vi "CRYO_LeakTest_tmp.vi"() -> ()   [LabVIEW 2017]
uses:
  USBData.lvclass
panel:
  in  "Stop Button":bool
  out "Cycle #":u32=37
  out "Time of Last Measurement":timestamp=timestamp(3679441672.677524 s since 1904-01-01)
  in  "wait (ms)":u32=1000
  in  "?":enum32{"CONFIG", "MEASUREMENT"}(tab)=enum."MEASUREMENT"
  in  "USBSettings":T1(array[cluster])=[{"Label"="0", "FileFormat"="%2.2f", "Physical CH"="Dev2/ai0", "ConversionType"={"Type"=enum."CC-10_LOG", "ConversionParameters"=[0.5, 9.0]}, "VoltageLimits"=[0.0, 10.0]}, {"Label"="1", "FileFormat"="%2.2f", "Physical CH"="Dev2/ai1", "ConversionType"={"Type"=enum."LeakDet_EXP", "ConversionParameters"=[0.0, 1.0]}, "VoltageLimits"=[0.0, 10.0]}, {"Label"="2", "FileFormat"="%2.2f", "Physical CH"="Dev2/ai2", "ConversionType"={"Type"=enum."LeakDet_Mantissa", "ConversionParameters"=[0.0, 1.0]}, "VoltageLimits"=[0.0, 10.0]}, {"Label"="3", "FileFormat"="%2.2f", "Physical CH"="Dev2/ai3", "ConversionType"={"Type"=enum."SimpleProp", "ConversionParameters"=[0.0, 1.0]}, "VoltageLimits"=[0.0, 10.0]}]
  in  "RUN identifier":string="TEST"
  in  "Base Path":path=path "C:/LabVIEW/DATA/TestData/TestSeries"
  in  "Activate":bool=TRUE
  out "error out":errorcluster
  in  "InstName":string="USB6210"
  out "Status":T2(ring)=enum."Waiting"
  out "Waveform Chart 2":dbl(graph)
  out "Waveform Chart":dbl(graph)
  out "LeakRate":dbl=7.334292864367354e-09 format="%_3e"
  in  "Take Screenshot! 1":bool
  in  "Screenshot suffix 1":string="Graph1"
  in  "log/linear 2":bool=TRUE
  in  "Plot in \nGraph2?":bool[](array[boolean])=[TRUE, TRUE, FALSE, FALSE, FALSE, FALSE]
  out "Graph 2":T3(graph)=[{"TimeArray"=[timestamp(3679441636.668932 s since 1904-01-01), timestamp(3679441637.669246 s since 1904-01-01), timestamp(3679441638.668856 s since 1904-01-01), timestamp(3679441639.6687136 s since 1904-01-01), timestamp(3679441640.6689286 s since 1904-01-01), timestamp(3679441641.669116 s since 1904-01-01), timestamp(3679441642.6704025 s since 1904-01-01), timestamp(3679441643.6717186 s since 1904-01-01), timestamp(3679441644.671928 s since 1904-01-01), timestamp(3679441645.6718183 s since 1904-01-01), timestamp(3679441646.6721153 s since 1904-01-01), timestamp(3679441647.672172 s since 1904-01-01), timestamp(3679441648.672178 s since 1904-01-01), timestamp(3679441649.672041 s since 1904-01-01), timestamp(3679441650.6726017 s since 1904-01-01), timestamp(3679441651.6730194 s since 1904-01-01), timestamp(3679441652.673001 s since 1904-01-01), timestamp(3679441653.6726832 s since 1904-01-01), timestamp(3679441654.673409 s since 1904-01-01), timestamp(3679441655.6734624 s since 1904-01-01), timestamp(3679441656.674424 s since 1904-01-01), timestamp(3679441657.675055 s since 1904-01-01), timestamp(3679441658.674728 s since 1904-01-01), timestamp(3679441659.6749954 s since 1904-01-01), timestamp(3679441660.6749263 s since 1904-01-01), timestamp(3679441661.6754694 s since 1904-01-01), timestamp(3679441662.6761866 s since 1904-01-01), timestamp(3679441663.675552 s since 1904-01-01), timestamp(3679441664.675677 s since 1904-01-01), timestamp(3679441665.6756015 s since 1904-01-01), timestamp(3679441666.675688 s since 1904-01-01), timestamp(3679441667.6754055 s since 1904-01-01), timestamp(3679441668.6766486 s since 1904-01-01), timestamp(3679441669.677348 s since 1904-01-01), timestamp(3679441670.6767225 s since 1904-01-01), timestamp(3679441671.6770015 s since 1904-01-01), timestamp(3679441672.677524 s since 1904-01-01)], "DataArray"=[70.50247496839857, -9.0, 4.487131051293313, 0.0]}, {"TimeArray"=[timestamp(3679441636.668932 s since 1904-01-01), timestamp(3679441637.669246 s since 1904-01-01), timestamp(3679441638.668856 s since 1904-01-01), timestamp(3679441639.6687136 s since 1904-01-01), timestamp(3679441640.6689286 s since 1904-01-01), timestamp(3679441641.669116 s since 1904-01-01), timestamp(3679441642.6704025 s since 1904-01-01), timestamp(3679441643.6717186 s since 1904-01-01), timestamp(3679441644.671928 s since 1904-01-01), timestamp(3679441645.6718183 s since 1904-01-01), timestamp(3679441646.6721153 s since 1904-01-01), timestamp(3679441647.672172 s since 1904-01-01), timestamp(3679441648.672178 s since 1904-01-01), timestamp(3679441649.672041 s since 1904-01-01), timestamp(3679441650.6726017 s since 1904-01-01), timestamp(3679441651.6730194 s since 1904-01-01), timestamp(3679441652.673001 s since 1904-01-01), timestamp(3679441653.6726832 s since 1904-01-01), timestamp(3679441654.673409 s since 1904-01-01), timestamp(3679441655.6734624 s since 1904-01-01), timestamp(3679441656.674424 s since 1904-01-01), timestamp(3679441657.675055 s since 1904-01-01), timestamp(3679441658.674728 s since 1904-01-01), timestamp(3679441659.6749954 s since 1904-01-01), timestamp(3679441660.6749263 s since 1904-01-01), timestamp(3679441661.6754694 s since 1904-01-01), timestamp(3679441662.6761866 s since 1904-01-01), timestamp(3679441663.675552 s since 1904-01-01), timestamp(3679441664.675677 s since 1904-01-01), timestamp(3679441665.6756015 s since 1904-01-01), timestamp(3679441666.675688 s since 1904-01-01), timestamp(3679441667.6754055 s since 1904-01-01), timestamp(3679441668.6766486 s since 1904-01-01), timestamp(3679441669.677348 s since 1904-01-01), timestamp(3679441670.6767225 s since 1904-01-01), timestamp(3679441671.6770015 s since 1904-01-01), timestamp(3679441672.677524 s since 1904-01-01)], "DataArray"=[70.45978396050337, -9.0, 5.396766437487628, 0.0]}, {"TimeArray"=[timestamp(3679441636.668932 s since 1904-01-01), timestamp(3679441637.669246 s since 1904-01-01), timestamp(3679441638.668856 s since 1904-01-01), timestamp(3679441639.6687136 s since 1904-01-01), timestamp(3679441640.6689286 s since 1904-01-01), timestamp(3679441641.669116 s since 1904-01-01), timestamp(3679441642.6704025 s since 1904-01-01), timestamp(3679441643.6717186 s since 1904-01-01), timestamp(3679441644.671928 s since 1904-01-01), timestamp(3679441645.6718183 s since 1904-01-01), timestamp(3679441646.6721153 s since 1904-01-01), timestamp(3679441647.672172 s since 1904-01-01), timestamp(3679441648.672178 s since 1904-01-01), timestamp(3679441649.672041 s since 1904-01-01), timestamp(3679441650.6726017 s since 1904-01-01), timestamp(3679441651.6730194 s since 1904-01-01), timestamp(3679441652.673001 s since 1904-01-01), timestamp(3679441653.6726832 s since 1904-01-01), timestamp(3679441654.673409 s since 1904-01-01), timestamp(3679441655.6734624 s since 1904-01-01), timestamp(3679441656.674424 s since 1904-01-01), timestamp(3679441657.675055 s since 1904-01-01), timestamp(3679441658.674728 s since 1904-01-01), timestamp(3679441659.6749954 s since 1904-01-01), timestamp(3679441660.6749263 s since 1904-01-01), timestamp(3679441661.6754694 s since 1904-01-01), timestamp(3679441662.6761866 s since 1904-01-01), timestamp(3679441663.675552 s since 1904-01-01), timestamp(3679441664.675677 s since 1904-01-01), timestamp(3679441665.6756015 s since 1904-01-01), timestamp(3679441666.675688 s since 1904-01-01), timestamp(3679441667.6754055 s since 1904-01-01), timestamp(3679441668.6766486 s since 1904-01-01), timestamp(3679441669.677348 s since 1904-01-01), timestamp(3679441670.6767225 s since 1904-01-01), timestamp(3679441671.6770015 s since 1904-01-01), timestamp(3679441672.677524 s since 1904-01-01)], "DataArray"=[70.11918514591878, -9.0, 6.016059802087263, 0.0]}, {"TimeArray"=[timestamp(3679441636.668932 s since 1904-01-01), timestamp(3679441637.669246 s since 1904-01-01), timestamp(3679441638.668856 s since 1904-01-01), timestamp(3679441639.6687136 s since 1904-01-01), timestamp(3679441640.6689286 s since 1904-01-01), timestamp(3679441641.669116 s since 1904-01-01), timestamp(3679441642.6704025 s since 1904-01-01), timestamp(3679441643.6717186 s since 1904-01-01), timestamp(3679441644.671928 s since 1904-01-01), timestamp(3679441645.6718183 s since 1904-01-01), timestamp(3679441646.6721153 s since 1904-01-01), timestamp(3679441647.672172 s since 1904-01-01), timestamp(3679441648.672178 s since 1904-01-01), timestamp(3679441649.672041 s since 1904-01-01), timestamp(3679441650.6726017 s since 1904-01-01), timestamp(3679441651.6730194 s since 1904-01-01), timestamp(3679441652.673001 s since 1904-01-01), timestamp(3679441653.6726832 s since 1904-01-01), timestamp(3679441654.673409 s since 1904-01-01), timestamp(3679441655.6734624 s since 1904-01-01), timestamp(3679441656.674424 s since 1904-01-01), timestamp(3679441657.675055 s since 1904-01-01), timestamp(3679441658.674728 s since 1904-01-01), timestamp(3679441659.6749954 s since 1904-01-01), timestamp(3679441660.6749263 s since 1904-01-01), timestamp(3679441661.6754694 s since 1904-01-01), timestamp(3679441662.6761866 s since 1904-01-01), timestamp(3679441663.675552 s since 1904-01-01), timestamp(3679441664.675677 s since 1904-01-01), timestamp(3679441665.6756015 s since 1904-01-01), timestamp(3679441666.675688 s since 1904-01-01), timestamp(3679441667.6754055 s since 1904-01-01), timestamp(3679441668.6766486 s since 1904-01-01), timestamp(3679441669.677348 s since 1904-01-01), timestamp(3679441670.6767225 s since 1904-01-01), timestamp(3679441671.6770015 s since 1904-01-01), timestamp(3679441672.677524 s since 1904-01-01)], "DataArray"=[75.51986553242087, -9.0, 6.43017264767335, 0.0]}, {"TimeArray"=[timestamp(3679441636.668932 s since 1904-01-01), timestamp(3679441637.669246 s since 1904-01-01), timestamp(3679441638.668856 s since 1904-01-01), timestamp(3679441639.6687136 s since 1904-01-01), timestamp(3679441640.6689286 s since 1904-01-01), timestamp(3679441641.669116 s since 1904-01-01), timestamp(3679441642.6704025 s since 1904-01-01), timestamp(3679441643.6717186 s since 1904-01-01), timestamp(3679441644.671928 s since 1904-01-01), timestamp(3679441645.6718183 s since 1904-01-01), timestamp(3679441646.6721153 s since 1904-01-01), timestamp(3679441647.672172 s since 1904-01-01), timestamp(3679441648.672178 s since 1904-01-01), timestamp(3679441649.672041 s since 1904-01-01), timestamp(3679441650.6726017 s since 1904-01-01), timestamp(3679441651.6730194 s since 1904-01-01), timestamp(3679441652.673001 s since 1904-01-01), timestamp(3679441653.6726832 s since 1904-01-01), timestamp(3679441654.673409 s since 1904-01-01), timestamp(3679441655.6734624 s since 1904-01-01), timestamp(3679441656.674424 s since 1904-01-01), timestamp(3679441657.675055 s since 1904-01-01), timestamp(3679441658.674728 s since 1904-01-01), timestamp(3679441659.6749954 s since 1904-01-01), timestamp(3679441660.6749263 s since 1904-01-01), timestamp(3679441661.6754694 s since 1904-01-01), timestamp(3679441662.6761866 s since 1904-01-01), timestamp(3679441663.675552 s since 1904-01-01), timestamp(3679441664.675677 s since 1904-01-01), timestamp(3679441665.6756015 s since 1904-01-01), timestamp(3679441666.675688 s since 1904-01-01), timestamp(3679441667.6754055 s since 1904-01-01), timestamp(3679441668.6766486 s since 1904-01-01), timestamp(3679441669.677348 s since 1904-01-01), timestamp(3679441670.6767225 s since 1904-01-01), timestamp(3679441671.6770015 s since 1904-01-01), timestamp(3679441672.677524 s since 1904-01-01)], "DataArray"=[72.7584215196649, -9.0, 6.711377973370896, 0.0]}, {"TimeArray"=[timestamp(3679441636.668932 s since 1904-01-01), timestamp(3679441637.669246 s since 1904-01-01), timestamp(3679441638.668856 s since 1904-01-01), timestamp(3679441639.6687136 s since 1904-01-01), timestamp(3679441640.6689286 s since 1904-01-01), timestamp(3679441641.669116 s since 1904-01-01), timestamp(3679441642.6704025 s since 1904-01-01), timestamp(3679441643.6717186 s since 1904-01-01), timestamp(3679441644.671928 s since 1904-01-01), timestamp(3679441645.6718183 s since 1904-01-01), timestamp(3679441646.6721153 s since 1904-01-01), timestamp(3679441647.672172 s since 1904-01-01), timestamp(3679441648.672178 s since 1904-01-01), timestamp(3679441649.672041 s since 1904-01-01), timestamp(3679441650.6726017 s since 1904-01-01), timestamp(3679441651.6730194 s since 1904-01-01), timestamp(3679441652.673001 s since 1904-01-01), timestamp(3679441653.6726832 s since 1904-01-01), timestamp(3679441654.673409 s since 1904-01-01), timestamp(3679441655.6734624 s since 1904-01-01), timestamp(3679441656.674424 s since 1904-01-01), timestamp(3679441657.675055 s since 1904-01-01), timestamp(3679441658.674728 s since 1904-01-01), timestamp(3679441659.6749954 s since 1904-01-01), timestamp(3679441660.6749263 s since 1904-01-01), timestamp(3679441661.6754694 s since 1904-01-01), timestamp(3679441662.6761866 s since 1904-01-01), timestamp(3679441663.675552 s since 1904-01-01), timestamp(3679441664.675677 s since 1904-01-01), timestamp(3679441665.6756015 s since 1904-01-01), timestamp(3679441666.675688 s since 1904-01-01), timestamp(3679441667.6754055 s since 1904-01-01), timestamp(3679441668.6766486 s since 1904-01-01), timestamp(3679441669.677348 s since 1904-01-01), timestamp(3679441670.6767225 s since 1904-01-01), timestamp(3679441671.6770015 s since 1904-01-01), timestamp(3679441672.677524 s since 1904-01-01)], "DataArray"=[4.487131051293314e-09, 5.396766437487628e-09, 6.016059802087263e-09, 6.430172647673351e-09, 6.711377973370896e-09, 6.899791063470254e-09, 7.023690049144573e-09, 7.123059208849688e-09, 7.183956553663248e-09, 7.2279525979897775e-09, 7.25754635696336e-09, 7.2743819199666565e-09, 7.285430259185793e-09, 7.2907571374582694e-09, 7.29884610085954e-09, 7.306737772921106e-09, 7.30930256649171e-09, 7.3202851443231995e-09, 7.326138135237289e-09, 7.323441813920113e-09, 7.328834456885956e-09, 7.325283203914373e-09, 7.331201958895281e-09, 7.326861538535115e-09, 7.330807375263062e-09, 7.33231994614466e-09, 7.3306758473074275e-09, 7.326664246703097e-09, 7.3291632766052906e-09, 7.335082031766526e-09, 7.332911821527113e-09, 7.3328460575291335e-09, 7.333174877285675e-09, 7.337844117606753e-09, 7.332451473872307e-09, 7.335279323589255e-09, 7.334292864367354e-09]}] caption="XY Graph"
  out "Graph 1":T4(graph)=[{"TimeArray"=[timestamp(3679441636.668932 s since 1904-01-01), timestamp(3679441637.669246 s since 1904-01-01), timestamp(3679441638.668856 s since 1904-01-01), timestamp(3679441639.6687136 s since 1904-01-01), timestamp(3679441640.6689286 s since 1904-01-01), timestamp(3679441641.669116 s since 1904-01-01), timestamp(3679441642.6704025 s since 1904-01-01), timestamp(3679441643.6717186 s since 1904-01-01), timestamp(3679441644.671928 s since 1904-01-01), timestamp(3679441645.6718183 s since 1904-01-01), timestamp(3679441646.6721153 s since 1904-01-01), timestamp(3679441647.672172 s since 1904-01-01), timestamp(3679441648.672178 s since 1904-01-01), timestamp(3679441649.672041 s since 1904-01-01), timestamp(3679441650.6726017 s since 1904-01-01), timestamp(3679441651.6730194 s since 1904-01-01), timestamp(3679441652.673001 s since 1904-01-01), timestamp(3679441653.6726832 s since 1904-01-01), timestamp(3679441654.673409 s since 1904-01-01), timestamp(3679441655.6734624 s since 1904-01-01), timestamp(3679441656.674424 s since 1904-01-01), timestamp(3679441657.675055 s since 1904-01-01), timestamp(3679441658.674728 s since 1904-01-01), timestamp(3679441659.6749954 s since 1904-01-01), timestamp(3679441660.6749263 s since 1904-01-01), timestamp(3679441661.6754694 s since 1904-01-01), timestamp(3679441662.6761866 s since 1904-01-01), timestamp(3679441663.675552 s since 1904-01-01), timestamp(3679441664.675677 s since 1904-01-01), timestamp(3679441665.6756015 s since 1904-01-01), timestamp(3679441666.675688 s since 1904-01-01), timestamp(3679441667.6754055 s since 1904-01-01), timestamp(3679441668.6766486 s since 1904-01-01), timestamp(3679441669.677348 s since 1904-01-01), timestamp(3679441670.6767225 s since 1904-01-01), timestamp(3679441671.6770015 s since 1904-01-01), timestamp(3679441672.677524 s since 1904-01-01)], "LDArray"=[70.50247496839857, -9.0, 4.487131051293313, 0.0]}, {"TimeArray"=[timestamp(3679441636.668932 s since 1904-01-01), timestamp(3679441637.669246 s since 1904-01-01), timestamp(3679441638.668856 s since 1904-01-01), timestamp(3679441639.6687136 s since 1904-01-01), timestamp(3679441640.6689286 s since 1904-01-01), timestamp(3679441641.669116 s since 1904-01-01), timestamp(3679441642.6704025 s since 1904-01-01), timestamp(3679441643.6717186 s since 1904-01-01), timestamp(3679441644.671928 s since 1904-01-01), timestamp(3679441645.6718183 s since 1904-01-01), timestamp(3679441646.6721153 s since 1904-01-01), timestamp(3679441647.672172 s since 1904-01-01), timestamp(3679441648.672178 s since 1904-01-01), timestamp(3679441649.672041 s since 1904-01-01), timestamp(3679441650.6726017 s since 1904-01-01), timestamp(3679441651.6730194 s since 1904-01-01), timestamp(3679441652.673001 s since 1904-01-01), timestamp(3679441653.6726832 s since 1904-01-01), timestamp(3679441654.673409 s since 1904-01-01), timestamp(3679441655.6734624 s since 1904-01-01), timestamp(3679441656.674424 s since 1904-01-01), timestamp(3679441657.675055 s since 1904-01-01), timestamp(3679441658.674728 s since 1904-01-01), timestamp(3679441659.6749954 s since 1904-01-01), timestamp(3679441660.6749263 s since 1904-01-01), timestamp(3679441661.6754694 s since 1904-01-01), timestamp(3679441662.6761866 s since 1904-01-01), timestamp(3679441663.675552 s since 1904-01-01), timestamp(3679441664.675677 s since 1904-01-01), timestamp(3679441665.6756015 s since 1904-01-01), timestamp(3679441666.675688 s since 1904-01-01), timestamp(3679441667.6754055 s since 1904-01-01), timestamp(3679441668.6766486 s since 1904-01-01), timestamp(3679441669.677348 s since 1904-01-01), timestamp(3679441670.6767225 s since 1904-01-01), timestamp(3679441671.6770015 s since 1904-01-01), timestamp(3679441672.677524 s since 1904-01-01)], "LDArray"=[70.45978396050337, -9.0, 5.396766437487628, 0.0]}, {"TimeArray"=[timestamp(3679441636.668932 s since 1904-01-01), timestamp(3679441637.669246 s since 1904-01-01), timestamp(3679441638.668856 s since 1904-01-01), timestamp(3679441639.6687136 s since 1904-01-01), timestamp(3679441640.6689286 s since 1904-01-01), timestamp(3679441641.669116 s since 1904-01-01), timestamp(3679441642.6704025 s since 1904-01-01), timestamp(3679441643.6717186 s since 1904-01-01), timestamp(3679441644.671928 s since 1904-01-01), timestamp(3679441645.6718183 s since 1904-01-01), timestamp(3679441646.6721153 s since 1904-01-01), timestamp(3679441647.672172 s since 1904-01-01), timestamp(3679441648.672178 s since 1904-01-01), timestamp(3679441649.672041 s since 1904-01-01), timestamp(3679441650.6726017 s since 1904-01-01), timestamp(3679441651.6730194 s since 1904-01-01), timestamp(3679441652.673001 s since 1904-01-01), timestamp(3679441653.6726832 s since 1904-01-01), timestamp(3679441654.673409 s since 1904-01-01), timestamp(3679441655.6734624 s since 1904-01-01), timestamp(3679441656.674424 s since 1904-01-01), timestamp(3679441657.675055 s since 1904-01-01), timestamp(3679441658.674728 s since 1904-01-01), timestamp(3679441659.6749954 s since 1904-01-01), timestamp(3679441660.6749263 s since 1904-01-01), timestamp(3679441661.6754694 s since 1904-01-01), timestamp(3679441662.6761866 s since 1904-01-01), timestamp(3679441663.675552 s since 1904-01-01), timestamp(3679441664.675677 s since 1904-01-01), timestamp(3679441665.6756015 s since 1904-01-01), timestamp(3679441666.675688 s since 1904-01-01), timestamp(3679441667.6754055 s since 1904-01-01), timestamp(3679441668.6766486 s since 1904-01-01), timestamp(3679441669.677348 s since 1904-01-01), timestamp(3679441670.6767225 s since 1904-01-01), timestamp(3679441671.6770015 s since 1904-01-01), timestamp(3679441672.677524 s since 1904-01-01)], "LDArray"=[70.11918514591878, -9.0, 6.016059802087263, 0.0]}, {"TimeArray"=[timestamp(3679441636.668932 s since 1904-01-01), timestamp(3679441637.669246 s since 1904-01-01), timestamp(3679441638.668856 s since 1904-01-01), timestamp(3679441639.6687136 s since 1904-01-01), timestamp(3679441640.6689286 s since 1904-01-01), timestamp(3679441641.669116 s since 1904-01-01), timestamp(3679441642.6704025 s since 1904-01-01), timestamp(3679441643.6717186 s since 1904-01-01), timestamp(3679441644.671928 s since 1904-01-01), timestamp(3679441645.6718183 s since 1904-01-01), timestamp(3679441646.6721153 s since 1904-01-01), timestamp(3679441647.672172 s since 1904-01-01), timestamp(3679441648.672178 s since 1904-01-01), timestamp(3679441649.672041 s since 1904-01-01), timestamp(3679441650.6726017 s since 1904-01-01), timestamp(3679441651.6730194 s since 1904-01-01), timestamp(3679441652.673001 s since 1904-01-01), timestamp(3679441653.6726832 s since 1904-01-01), timestamp(3679441654.673409 s since 1904-01-01), timestamp(3679441655.6734624 s since 1904-01-01), timestamp(3679441656.674424 s since 1904-01-01), timestamp(3679441657.675055 s since 1904-01-01), timestamp(3679441658.674728 s since 1904-01-01), timestamp(3679441659.6749954 s since 1904-01-01), timestamp(3679441660.6749263 s since 1904-01-01), timestamp(3679441661.6754694 s since 1904-01-01), timestamp(3679441662.6761866 s since 1904-01-01), timestamp(3679441663.675552 s since 1904-01-01), timestamp(3679441664.675677 s since 1904-01-01), timestamp(3679441665.6756015 s since 1904-01-01), timestamp(3679441666.675688 s since 1904-01-01), timestamp(3679441667.6754055 s since 1904-01-01), timestamp(3679441668.6766486 s since 1904-01-01), timestamp(3679441669.677348 s since 1904-01-01), timestamp(3679441670.6767225 s since 1904-01-01), timestamp(3679441671.6770015 s since 1904-01-01), timestamp(3679441672.677524 s since 1904-01-01)], "LDArray"=[75.51986553242087, -9.0, 6.43017264767335, 0.0]}, {"TimeArray"=[timestamp(3679441636.668932 s since 1904-01-01), timestamp(3679441637.669246 s since 1904-01-01), timestamp(3679441638.668856 s since 1904-01-01), timestamp(3679441639.6687136 s since 1904-01-01), timestamp(3679441640.6689286 s since 1904-01-01), timestamp(3679441641.669116 s since 1904-01-01), timestamp(3679441642.6704025 s since 1904-01-01), timestamp(3679441643.6717186 s since 1904-01-01), timestamp(3679441644.671928 s since 1904-01-01), timestamp(3679441645.6718183 s since 1904-01-01), timestamp(3679441646.6721153 s since 1904-01-01), timestamp(3679441647.672172 s since 1904-01-01), timestamp(3679441648.672178 s since 1904-01-01), timestamp(3679441649.672041 s since 1904-01-01), timestamp(3679441650.6726017 s since 1904-01-01), timestamp(3679441651.6730194 s since 1904-01-01), timestamp(3679441652.673001 s since 1904-01-01), timestamp(3679441653.6726832 s since 1904-01-01), timestamp(3679441654.673409 s since 1904-01-01), timestamp(3679441655.6734624 s since 1904-01-01), timestamp(3679441656.674424 s since 1904-01-01), timestamp(3679441657.675055 s since 1904-01-01), timestamp(3679441658.674728 s since 1904-01-01), timestamp(3679441659.6749954 s since 1904-01-01), timestamp(3679441660.6749263 s since 1904-01-01), timestamp(3679441661.6754694 s since 1904-01-01), timestamp(3679441662.6761866 s since 1904-01-01), timestamp(3679441663.675552 s since 1904-01-01), timestamp(3679441664.675677 s since 1904-01-01), timestamp(3679441665.6756015 s since 1904-01-01), timestamp(3679441666.675688 s since 1904-01-01), timestamp(3679441667.6754055 s since 1904-01-01), timestamp(3679441668.6766486 s since 1904-01-01), timestamp(3679441669.677348 s since 1904-01-01), timestamp(3679441670.6767225 s since 1904-01-01), timestamp(3679441671.6770015 s since 1904-01-01), timestamp(3679441672.677524 s since 1904-01-01)], "LDArray"=[72.7584215196649, -9.0, 6.711377973370896, 0.0]}, {"TimeArray"=[timestamp(3679441636.668932 s since 1904-01-01), timestamp(3679441637.669246 s since 1904-01-01), timestamp(3679441638.668856 s since 1904-01-01), timestamp(3679441639.6687136 s since 1904-01-01), timestamp(3679441640.6689286 s since 1904-01-01), timestamp(3679441641.669116 s since 1904-01-01), timestamp(3679441642.6704025 s since 1904-01-01), timestamp(3679441643.6717186 s since 1904-01-01), timestamp(3679441644.671928 s since 1904-01-01), timestamp(3679441645.6718183 s since 1904-01-01), timestamp(3679441646.6721153 s since 1904-01-01), timestamp(3679441647.672172 s since 1904-01-01), timestamp(3679441648.672178 s since 1904-01-01), timestamp(3679441649.672041 s since 1904-01-01), timestamp(3679441650.6726017 s since 1904-01-01), timestamp(3679441651.6730194 s since 1904-01-01), timestamp(3679441652.673001 s since 1904-01-01), timestamp(3679441653.6726832 s since 1904-01-01), timestamp(3679441654.673409 s since 1904-01-01), timestamp(3679441655.6734624 s since 1904-01-01), timestamp(3679441656.674424 s since 1904-01-01), timestamp(3679441657.675055 s since 1904-01-01), timestamp(3679441658.674728 s since 1904-01-01), timestamp(3679441659.6749954 s since 1904-01-01), timestamp(3679441660.6749263 s since 1904-01-01), timestamp(3679441661.6754694 s since 1904-01-01), timestamp(3679441662.6761866 s since 1904-01-01), timestamp(3679441663.675552 s since 1904-01-01), timestamp(3679441664.675677 s since 1904-01-01), timestamp(3679441665.6756015 s since 1904-01-01), timestamp(3679441666.675688 s since 1904-01-01), timestamp(3679441667.6754055 s since 1904-01-01), timestamp(3679441668.6766486 s since 1904-01-01), timestamp(3679441669.677348 s since 1904-01-01), timestamp(3679441670.6767225 s since 1904-01-01), timestamp(3679441671.6770015 s since 1904-01-01), timestamp(3679441672.677524 s since 1904-01-01)], "LDArray"=[4.487131051293314e-09, 5.396766437487628e-09, 6.016059802087263e-09, 6.430172647673351e-09, 6.711377973370896e-09, 6.899791063470254e-09, 7.023690049144573e-09, 7.123059208849688e-09, 7.183956553663248e-09, 7.2279525979897775e-09, 7.25754635696336e-09, 7.2743819199666565e-09, 7.285430259185793e-09, 7.2907571374582694e-09, 7.29884610085954e-09, 7.306737772921106e-09, 7.30930256649171e-09, 7.3202851443231995e-09, 7.326138135237289e-09, 7.323441813920113e-09, 7.328834456885956e-09, 7.325283203914373e-09, 7.331201958895281e-09, 7.326861538535115e-09, 7.330807375263062e-09, 7.33231994614466e-09, 7.3306758473074275e-09, 7.326664246703097e-09, 7.3291632766052906e-09, 7.335082031766526e-09, 7.332911821527113e-09, 7.3328460575291335e-09, 7.333174877285675e-09, 7.337844117606753e-09, 7.332451473872307e-09, 7.335279323589255e-09, 7.334292864367354e-09]}] caption="XY Graph"
  out "LastData":dbl[](array[numeric])=[76.85813213557458, -9.0, 7.334292864367354, 0.0, 7.334292864367354e-09]
  out "AllSeries":string[](array[string])=["0", "1", "2", "3", "LaekDet_FULL"]
  in  "Plot in \nGraph1?":bool[](array[boolean])=[FALSE, TRUE, FALSE, FALSE, TRUE, FALSE]
  in  "log/linear 1":bool
  in  "Take Screenshot! 2":bool
  in  "Screenshot suffix 2":string="Graph2"
  # "GLOBAL STATUS/CONTROL"
  # "USB6210 Settings"
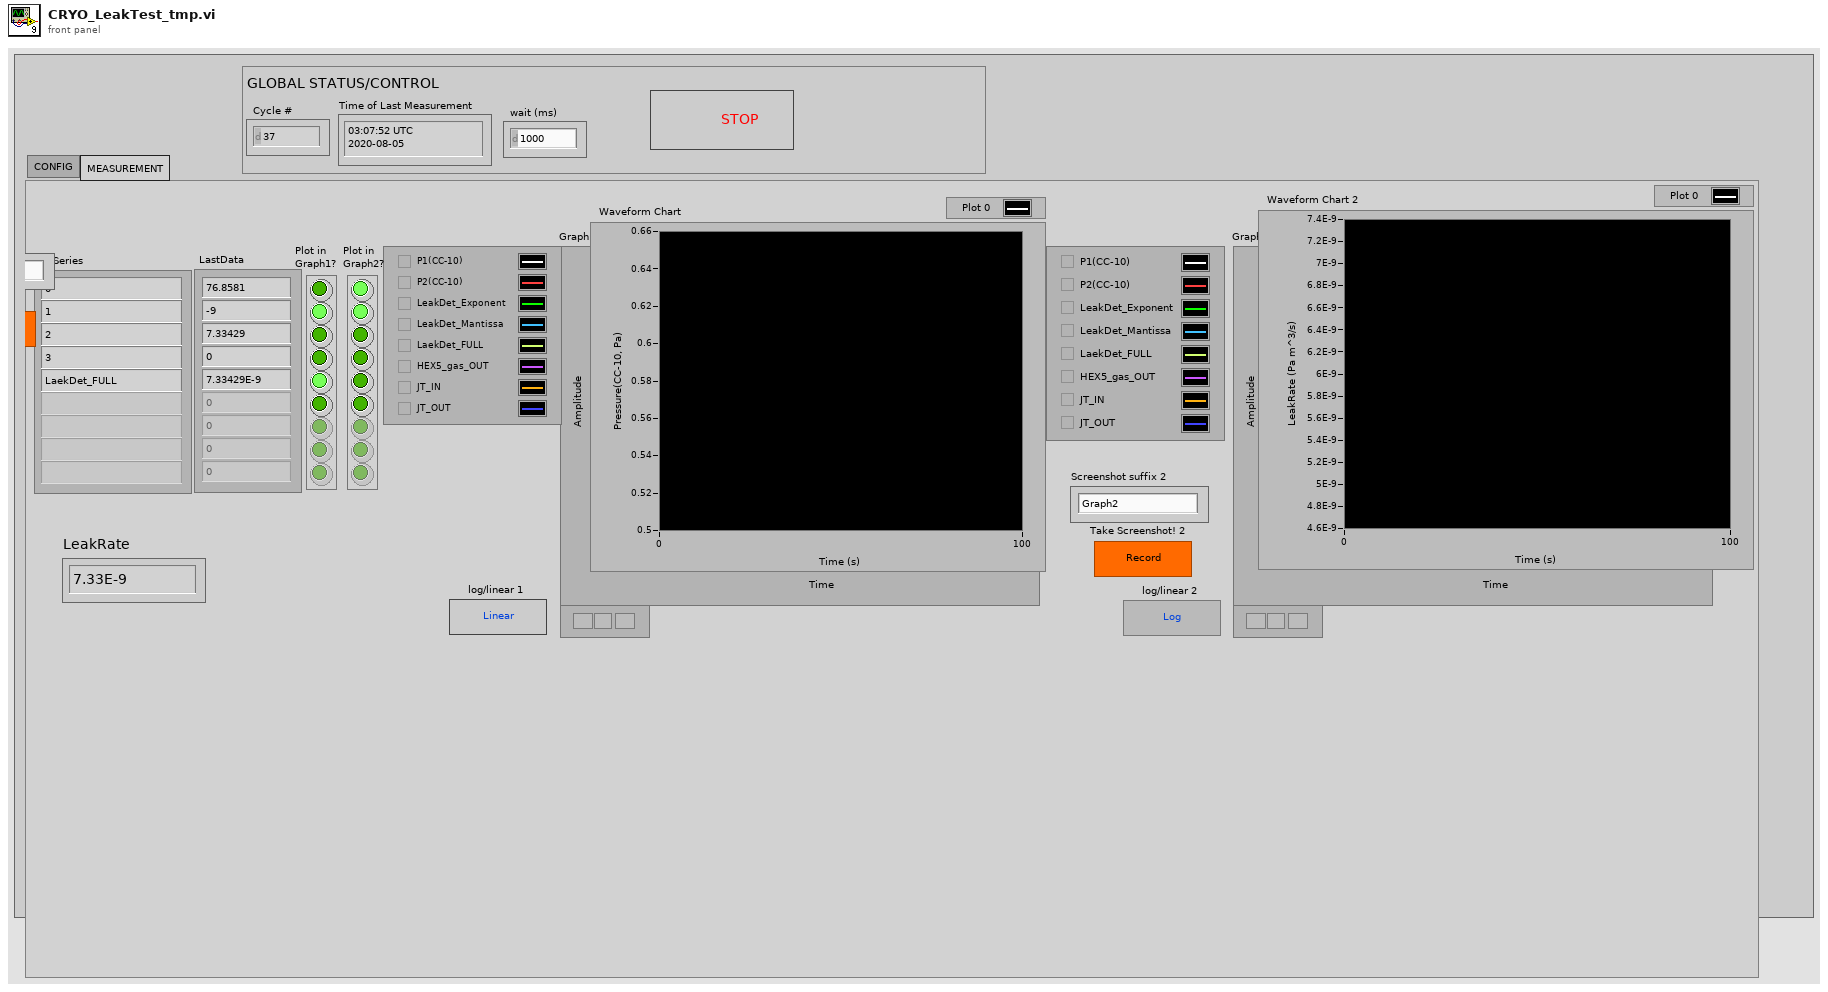
[diagram p1: front panel]
types:
  T1 = cluster{"Label":string, "FileFormat":string, "Physical CH":tag, "ConversionType":cluster{"Type":enum16{"SimpleProp", "CC-10_COMBINED", "CC-10_LOG", "LeakDet_EXP", "LeakDet_Mantissa", "Baratron"}, "ConversionParameters":dbl[]}, "VoltageLimits":dbl[]}[]
  T2 = enum16{"Intialized", "Waiting", "Measuring", "Terminated"}
  T3 = cluster{"TimeArray":timestamp[], "DataArray":dbl[]}[]
  T4 = cluster{"TimeArray":timestamp[], "LDArray":dbl[]}[]
  T5 = cluster{"TimeArray":timestamp[], "DataArrayConv":dbl[]}[]
  T6 = cluster{"IndexArray":i64[], "TimeArray":timestamp[], "DataArrayRaw":dbl[][], "DataArrayConv":dbl[][], "LDArray":dbl[]}
  T7 = cluster{"InstName":string, "Active?":bool, "Status":enum16{"Intialized", "Waiting", "Measuring", "Terminated"}, "Labels":string[], "LabelLD":string, "FileFormat":string[], "FileFormatLD":string, "ReadLeakDet?":bool}
  T8 = cluster{"TimeArray":timestamp[], "DataArrayConv":dbl[]}
  T9 = cluster{"TimeArray":timestamp[], "LDArray":dbl[]}
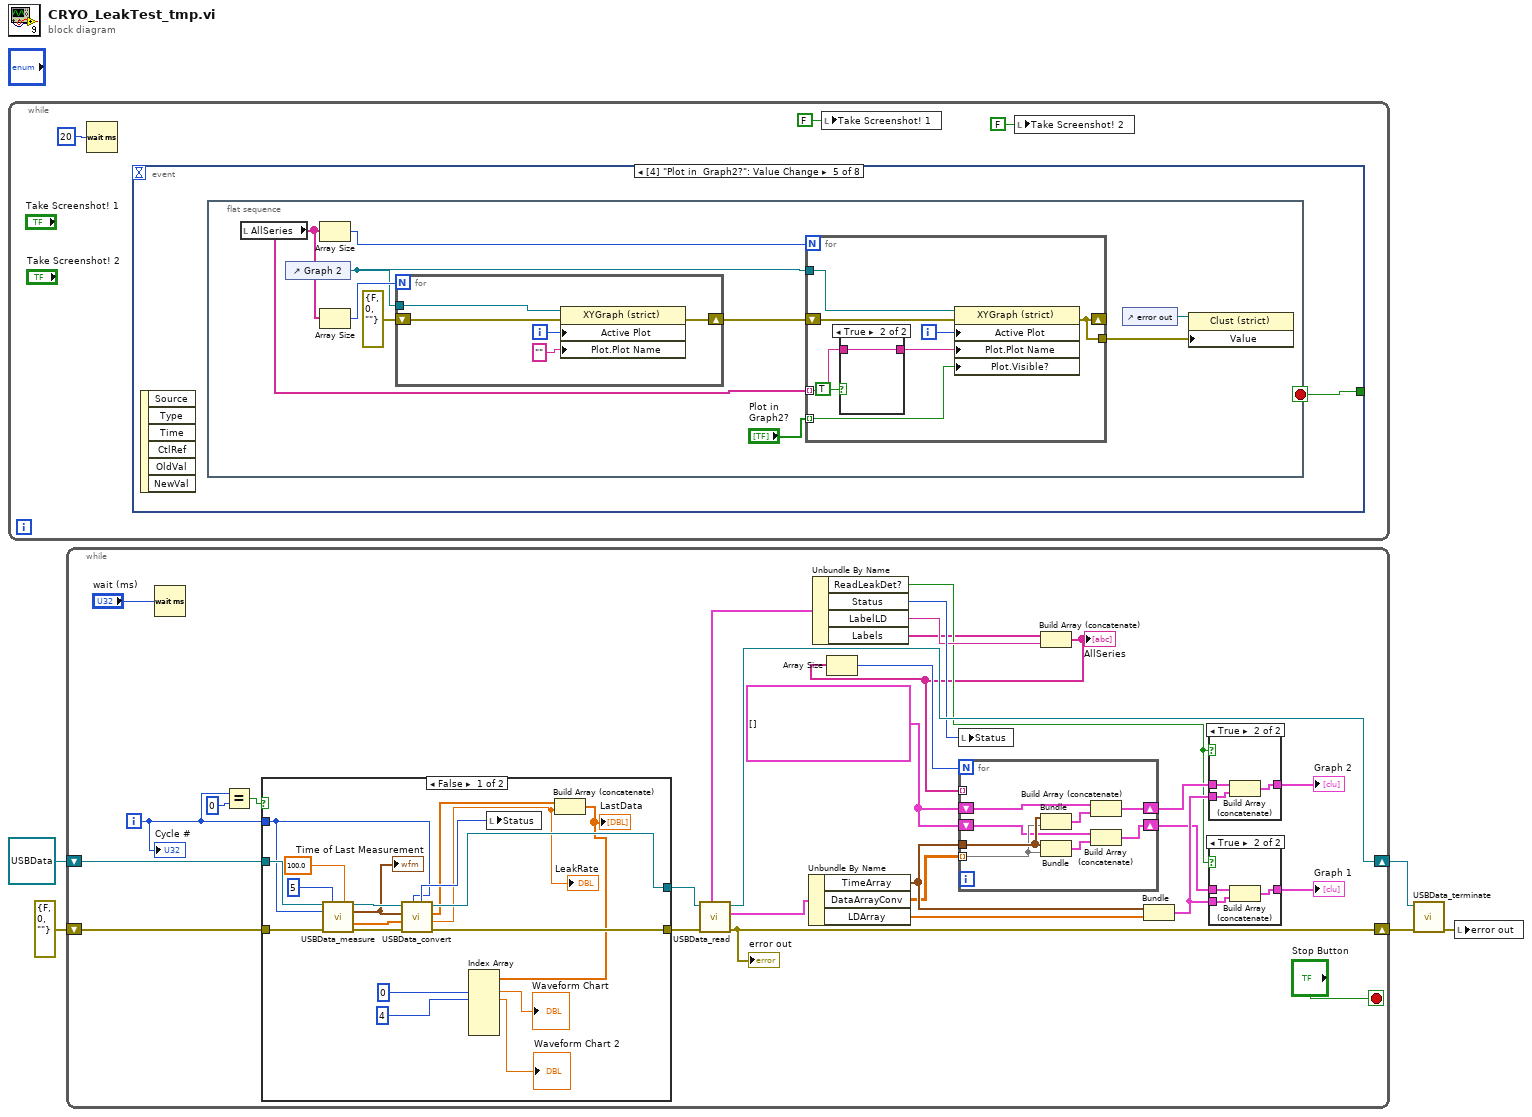
[diagram p0: block diagram]
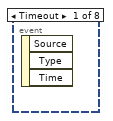
[diagram p2: hidden frame]
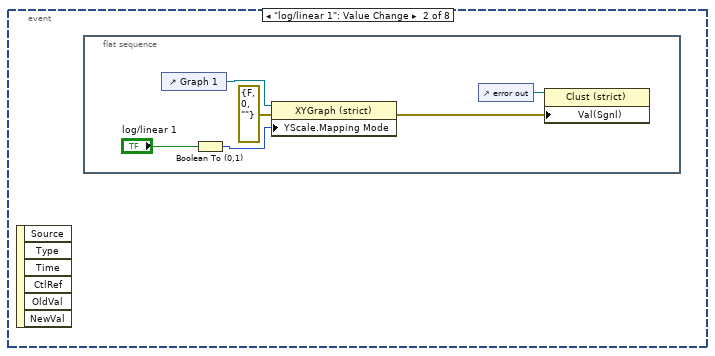
[diagram p3: hidden frame]
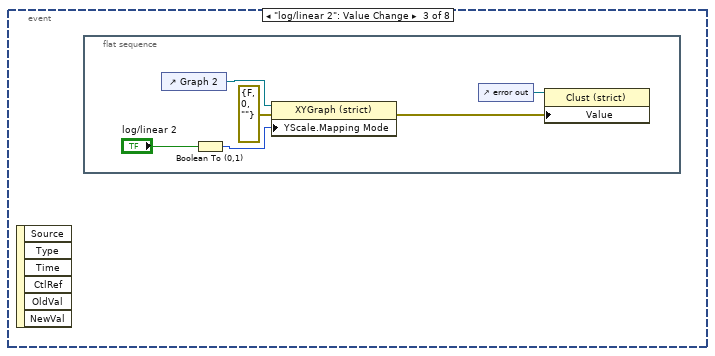
[diagram p4: hidden frame]
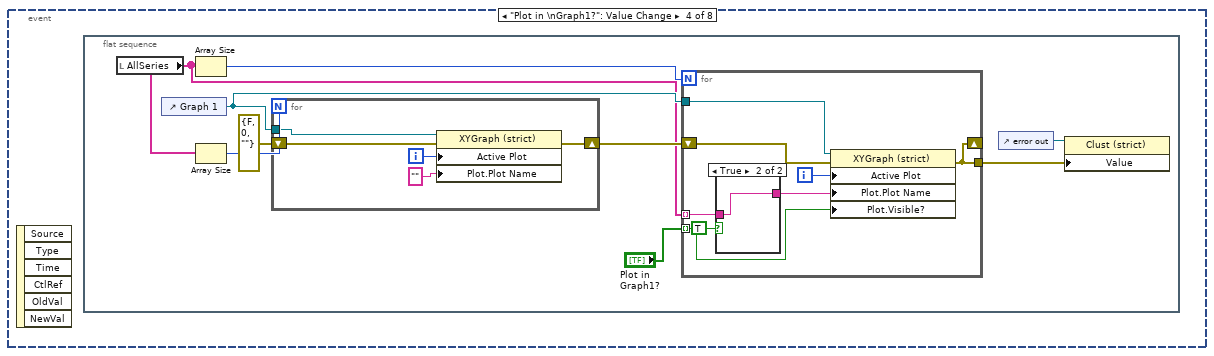
[diagram p5: hidden frame]
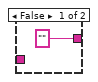
[diagram p6: hidden frame]
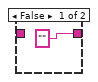
[diagram p7: hidden frame]
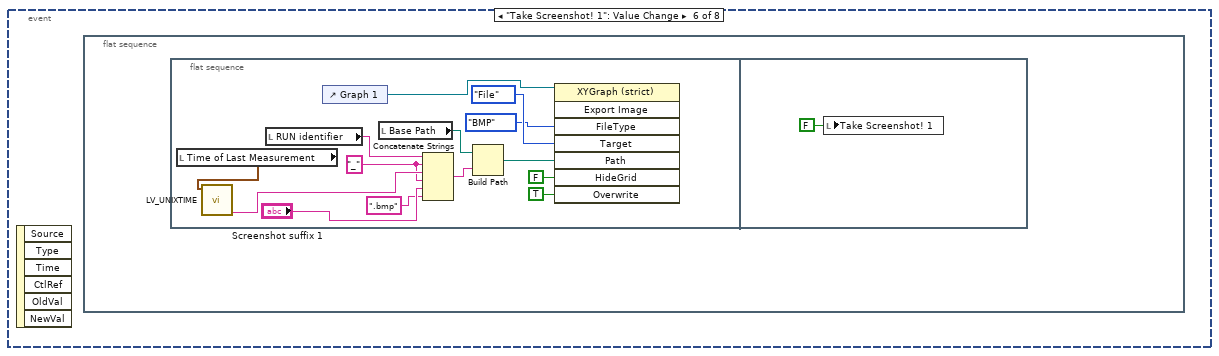
[diagram p8: hidden frame]
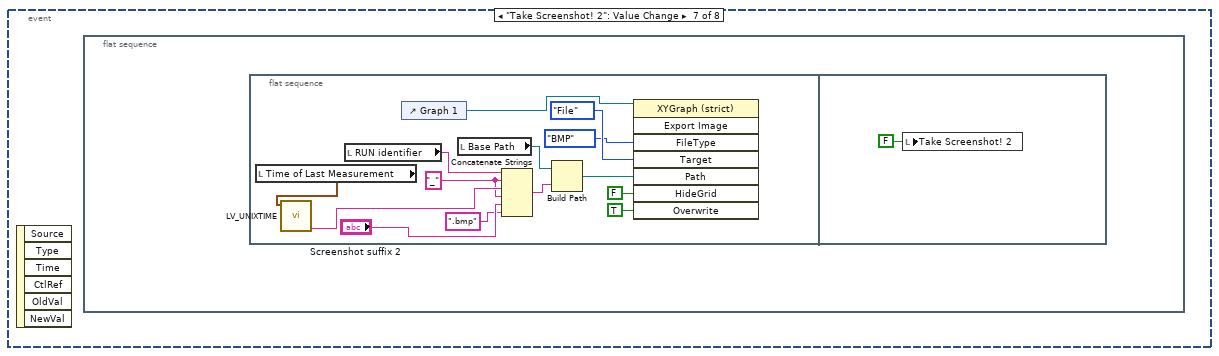
[diagram p9: hidden frame]
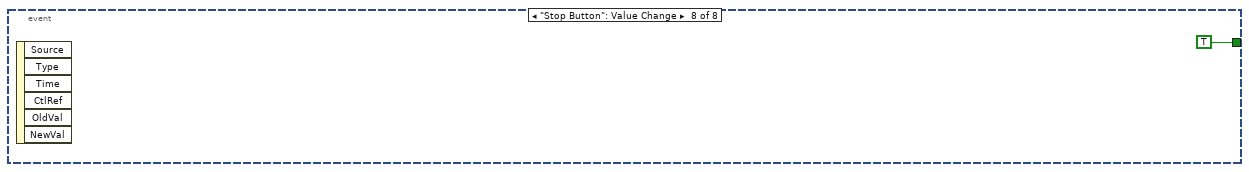
[diagram p10: hidden frame]
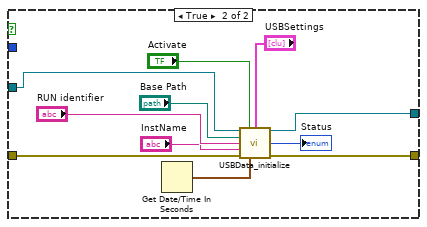
[diagram p13: hidden frame]
diagram:
  n1 = while {
    stop <- w8 stop-if-true
    n2 = Wait (ms)(milliseconds to wait=u32 20) -> ()  [unwired: 1 out]
    n3 = event shown="[4] \"Plot in  Graph2?\": Value Change" {
      selector: _ -> [_ _ _ _ _ _ _ _]
      dyn-events: _ -> [_ _ _ _ _ _ _ _]
      timeout: _ -> [_ _ _ _ _ _ _ _]
      tunnel: [_ _ _ _ _ _ _ TRUE] -> w8
      event Timeout {
        n4 = event-data() -> ()  [unwired: 1 in, 3 out]
      }
      event "log/linear 1": Value Change {
        n5 = event-data() -> ()  [unwired: 1 in, 6 out]
        n6 = flat-sequence {
          frame #0 {
            n7 = control-ref of="Graph 1"() -> (w13:refnum<vi>)
            n8 = Boolean To (0,1)(Boolean="log/linear 1") -> (0, 1=w14:i16)
            n9 = property class="XYGraph (strict)"(reference=w13, error in=errorcluster {"status"=FALSE, "code"=0, "source"=""} ("error in (no error)"), "YScale.Mapping Mode"=w14) -> (error out=w11:errorcluster)  [unwired: 1 out]
            n10 = control-ref of="error out"() -> (w12:refnum<vi>)
            n11 = property class="Clust (strict)"(reference=w12, "Val(Sgnl)"=w11) -> ()  [unwired: 1 in, 2 out]
          }
        }
      }
      event "log/linear 2": Value Change {
        n12 = event-data() -> ()  [unwired: 1 in, 6 out]
        n13 = flat-sequence {
          frame #0 {
            n14 = control-ref of="Graph 2"() -> (w17:refnum<vi>)
            n15 = Boolean To (0,1)(Boolean="log/linear 2") -> (0, 1=w20:i16)
            n16 = property class="XYGraph (strict)"(reference=w17, error in=errorcluster {"status"=FALSE, "code"=0, "source"=""} ("error in (no error)"), "YScale.Mapping Mode"=w20) -> (error out=w19:errorcluster)  [unwired: 1 out]
            n17 = control-ref of="error out"() -> (w16:refnum<vi>)
            n18 = property class="Clust (strict)"(reference=w16, "Value"=w19) -> ()  [unwired: 1 in, 2 out]
          }
        }
      }
      event "Plot in \nGraph1?": Value Change {
        n19 = event-data() -> ()  [unwired: 1 in, 6 out]
        n20 = flat-sequence {
          frame #0 {
            n21 = local read "AllSeries"() -> (w23:string[])
            n22 = control-ref of="Graph 1"() -> (w27:refnum<vi>)
            n23 = Array Size(array=w23) -> (size(s)=w28:i32)
            n24 = Array Size(array=w23) -> (size(s)=w29:i32)
            n25 = for {
              N: w29 -> [_]
              tunnel: w27 -> [w43]
              shift-right: [w41] -> w25
              shift-left: errorcluster {"status"=FALSE, "code"=0, "source"=""} ("error in (no error)") -> [w42]
              i -> [w45]
              n26 = property class="XYGraph (strict)"(reference=w43, error in=w42, "Active Plot"=w45, "Plot.Plot Name"="") -> (error out=w41:errorcluster)  [unwired: 1 out]
            }
            n27 = for {
              N: w28 -> [_]
              tunnel: w27 -> [w37]
              shift-right: [w35] -> _
              shift-left: w25 -> [w36]
              tunnel: [w35] -> w24
              tunnel: "Plot in \nGraph1?" -> [w32] mode=indexing
              tunnel: w23 -> [w33] mode=indexing
              i -> [w38]
              n28 = case shown="True" TRUE {
                tunnel: ["" ("Plot.Plot Name") w40] -> w34
                tunnel: w33 -> [_ w40]
                frame False {
                }
                frame True {
                }
              }
              n29 = property class="XYGraph (strict)"(reference=w37, error in=w36, "Active Plot"=w38, "Plot.Plot Name"=w34, "Plot.Visible?"=w32) -> (error out=w35:errorcluster)  [unwired: 1 out]
            }
            n30 = control-ref of="error out"() -> (w30:refnum<vi>)
            n31 = property class="Clust (strict)"(reference=w30, "Value"=w24) -> ()  [unwired: 1 in, 2 out]
          }
        }
      }
      event "Plot in \nGraph2?": Value Change {
        n32 = event-data() -> ()  [unwired: 1 in, 6 out]
        n33 = flat-sequence {
          frame #0 {
            n34 = local read "AllSeries"() -> (w48:string[])
            n35 = control-ref of="Graph 2"() -> (w46:refnum<vi>)
            n36 = Array Size(array=w48) -> (size(s)=w52:i32)
            n37 = Array Size(array=w48) -> (size(s)=w53:i32)
            n38 = for {
              N: w53 -> [_]
              shift-right: [w66] -> w50
              shift-left: errorcluster {"status"=FALSE, "code"=0, "source"=""} ("error in (no error)") -> [w67]
              tunnel: w46 -> [w65]
              i -> [w69]
              n39 = property class="XYGraph (strict)"(reference=w65, error in=w67, "Active Plot"=w69, "Plot.Plot Name"="") -> (error out=w66:errorcluster)  [unwired: 1 out]
            }
            n40 = for {
              N: w52 -> [_]
              shift-right: [w60] -> _
              shift-left: w50 -> [w61]
              tunnel: [w60] -> w49
              tunnel: w48 -> [w58] mode=indexing
              tunnel: "Plot in \nGraph2?" -> [w57] mode=indexing
              tunnel: w46 -> [w56]
              i -> [w62]
              n41 = case shown="True" TRUE {
                tunnel: ["" ("Plot.Plot Name") w64] -> w59
                tunnel: w58 -> [_ w64]
                frame False {
                }
                frame True {
                }
              }
              n42 = property class="XYGraph (strict)"(reference=w56, error in=w61, "Active Plot"=w62, "Plot.Plot Name"=w59, "Plot.Visible?"=w57) -> (error out=w60:errorcluster)  [unwired: 1 out]
            }
            n43 = control-ref of="error out"() -> (w54:refnum<vi>)
            n44 = property class="Clust (strict)"(reference=w54, "Value"=w49) -> ()  [unwired: 1 in, 2 out]
          }
        }
      }
      event "Take Screenshot! 1": Value Change {
        n45 = event-data() -> ()  [unwired: 1 in, 6 out]
        n46 = flat-sequence {
          frame #0 {
            n47 = flat-sequence {
              frame #0 {
                w72 = "_" ("string")
                n48 = local read "Time of Last Measurement"() -> (w74:timestamp)
                n49 = call "LV_UNIXTIME.vi"("current time"=w74) -> ("date/time string"=w73:string)  [unwired: 9 in, 1 out]
                n50 = local read "RUN identifier"() -> (w77:string)
                n51 = control-ref of="Graph 1"() -> (w75:refnum<vi>)
                n52 = local read "Base Path"() -> (w78:path)
                n53 = Concatenate Strings(w77, w72, w73, w72, "Screenshot suffix 1", ".bmp" ("string")) -> (w83:string)
                n54 = Build Path(base path=w78, name or relative path=w83) -> (appended path=w82:path)
                n55 = invoke on="Invoke Node" class="XYGraph (strict)" method="Export Image"(reference=w75, "FileType"=enum32{"BMP", "EPS", "EMF", "PICT"}."BMP" ("File Type"), "Target"=enum32{"File", "Clipboard"}."File", "Path"=w82, "HideGrid"=FALSE ("Hide Grid"), "Overwrite"=TRUE ("Always Overwrite")) -> ()  [unwired: 2 in, 8 out]
              }
              frame #1 {
                n56 = local write "Take Screenshot! 1"(FALSE ("Take Screenshot! 1")) -> ()
              }
            }
          }
        }
      }
      event "Take Screenshot! 2": Value Change {
        n57 = event-data() -> ()  [unwired: 1 in, 6 out]
        n58 = flat-sequence {
          frame #0 {
            n59 = flat-sequence {
              frame #0 {
                w87 = "_" ("string")
                n60 = local read "Time of Last Measurement"() -> (w89:timestamp)
                n61 = call "LV_UNIXTIME.vi"("current time"=w89) -> ("date/time string"=w88:string)  [unwired: 9 in, 1 out]
                n62 = local read "RUN identifier"() -> (w92:string)
                n63 = control-ref of="Graph 1"() -> (w90:refnum<vi>)
                n64 = local read "Base Path"() -> (w93:path)
                n65 = Concatenate Strings(w92, w87, w88, w87, "Screenshot suffix 2", ".bmp" ("string")) -> (w98:string)
                n66 = Build Path(base path=w93, name or relative path=w98) -> (appended path=w97:path)
                n67 = invoke on="Invoke Node" class="XYGraph (strict)" method="Export Image"(reference=w90, "FileType"=enum32{"BMP", "EPS", "EMF", "PICT"}."BMP" ("File Type"), "Target"=enum32{"File", "Clipboard"}."File", "Path"=w97, "HideGrid"=FALSE ("Hide Grid"), "Overwrite"=TRUE ("Always Overwrite")) -> ()  [unwired: 2 in, 8 out]
              }
              frame #1 {
                n68 = local write "Take Screenshot! 2"(FALSE ("Take Screenshot! 1")) -> ()
              }
            }
          }
        }
      }
      event "Stop Button": Value Change {
        n69 = event-data() -> ()  [unwired: 1 in, 6 out]
      }
    }
    n70 = local write "Take Screenshot! 1"(FALSE ("Take Screenshot! 1")) -> ()
    n71 = local write "Take Screenshot! 2"(FALSE ("Take Screenshot! 1")) -> ()
  }
  n72 = while {
    shift-right: [w122] -> w3
    shift-left: refnum<class "USBData.lvclass"> refnum ("USBData.lvclass") -> [w125]
    shift-right: [w120] -> w2
    shift-left: errorcluster {"status"=FALSE, "code"=0, "source"=""} ("error in (no error)") -> [w124]
    i -> [w103]
    stop <- "Stop Button" stop-if-true
    w108 = T5 [] ("appended array")
    n73 = Wait (ms)(milliseconds to wait="wait (ms)") -> ()  [unwired: 1 out]
    n74 = Equal?(x=w103, y=0) -> (x = y?=w126:bool)
    n75 = case shown="False" w126 {
      tunnel: w125 -> [w163 w174]
      tunnel: [w155 w168] -> w123
      tunnel: w124 -> [w157 w167]
      tunnel: [w156 w166] -> w121
      tunnel: w103 -> [w152 _]
      frame False {
        n76 = call-dynamic "USBData_measure.vi"("USBData in"=w163, "DAQ sample #"=i64 5, "DAQ timeout"=100.0 ("DAQ timeout (def: 100)"), "MeasurementIndex"=w152, "error in (no error)"=w157) -> ("USBData out"=w162:refnum<class "USBData.lvclass">, "TimeMeasuremeent"=w159:timestamp, "LastDataAcquired"=w153:dbl[], "error out"=w158:errorcluster)  [unwired: 4 in, 3 out]
        "Time of Last Measurement" <- w159
        n77 = call-dynamic "USBData_convert.vi"("MeasurementIndex"=w152, "error in (no error)"=w158, "LastDataAcquired"=w153, "TimeMeasuremeent"=w159, "USBData in"=w162) -> ("error out"=w156:errorcluster, "LeakDet_FULL"=w150:dbl, "LastDataonverted"=w151:dbl[], "USBData out"=w155:refnum<class "USBData.lvclass">, "Status"=w154:T2)  [unwired: 2 in]
        "LeakRate" <- w150
        n78 = local write "Status"(w154) -> ()
        n79 = Build Array (concatenate)(w151, w150) -> (w149:dbl[])
        "LastData" <- w149
        n80 = Index Array(array=w149, index #1=0 ("index"), index #2=4 ("index")) -> (element #1=→"Waveform Chart":dbl, element #2=→"Waveform Chart 2":dbl)  [unwired: 4 in, 4 out]
      }
      frame True {
        n81 = Get Date/Time In Seconds() -> (seconds since 1Jan1904=w169:timestamp)
        n82 = call-dynamic "USBData_initialize.vi"("USBData in"=w174, "Activate?"="Activate", "SeriesSetting"="USBSettings", "BasePath"="Base Path", "RunName"="RUN identifier", "InstName"="InstName", "error in (no error)"=w167, "RUN start time"=w169) -> ("USBData out"=w168:refnum<class "USBData.lvclass">, "Status"=→"Status":T2, "error out"=w166:errorcluster)  [unwired: 3 in, 2 out]
      }
    }
    n83 = call "USBData_read.vi"("error in (no error)"=w121, "USBData in"=w123) -> ("error out"=w120:errorcluster, "Data"=w119:T6, "USBData out"=w122:refnum<class "USBData.lvclass">, "Basic"=w117:T7)  [unwired: 2 in, 2 out]
    "error out" <- w120
    n84 = Unbundle By Name(w119) -> ("TimeArray"=w118:timestamp[], "DataArrayConv"=w111:dbl[][], "LDArray"=w110:dbl[])
    n85 = Unbundle By Name(w117) -> ("ReadLeakDet?"=w105:bool, "Status"=w116:T2, "LabelLD"=w115:string, "Labels"=w104:string[])
    n86 = local write "Status"(w116) -> ()
    n87 = Build Array (concatenate)(w104, w115) -> (w101:string[])
    "AllSeries" <- w101
    n88 = Array Size(array=w101) -> (size(s)=w112:i32)
    n89 = for {
      N: w112 -> [_]
      tunnel: w111 -> [w143] mode=indexing
      tunnel: w118 -> [w144]
      tunnel: w101 -> [_] mode=indexing
      shift-right: [w140] -> w114
      shift-left: w108 -> [w139]
      shift-right: [w141] -> w109
      shift-left: w108 -> [w142]
      n90 = Bundle("TimeArray"=w144, "DataArrayConv"=w143) -> (w137:T8)  [unwired: 1 in]
      n91 = Bundle("TimeArray"=w144, "DataArrayConv"=w143) -> (w138:T8)  [unwired: 1 in]
      n92 = Build Array (concatenate)(w139, w137) -> (w140:T5)
      n93 = Build Array (concatenate)(w142, w138) -> (w141:T5)
    }
    n94 = Bundle("TimeArray"=w118, "LDArray"=w110) -> (w113:T9)  [unwired: 1 in]
    n95 = case shown="True" w105 {
      tunnel: [w129 w132] -> w106
      tunnel: w114 -> [w129 w131]
      tunnel: w113 -> [_ w130]
      frame False {
      }
      frame True {
        n96 = Build Array (concatenate)(w131, w130) -> (w132:T4)
      }
    }
    "Graph 2" <- w106
    n97 = case shown="True" w105 {
      tunnel: w113 -> [_ w136]
      tunnel: [w133 w135] -> w107
      tunnel: w109 -> [w133 w134]
      frame False {
      }
      frame True {
        n98 = Build Array (concatenate)(w134, w136) -> (w135:T4)
      }
    }
    "Graph 1" <- w107
    "Cycle #" <- w103
  }
  n99 = call-dynamic "USBData_terminate.vi"("error in (no error)"=w2, "USBData in"=w3) -> ("error out"=w1:errorcluster)  [unwired: 8 in, 1 out]
  n100 = local write "error out"(w1) -> ()
